vi "art联动采集V4.7(定点后行扫的方案).vi"() -> ()   [LabVIEW 2016]
uses:
  <vilib>/Instr/_visa.llb/VISA Configure Serial Port (Instr).vi
  <vilib>/Utility/file.llb/Write Delimited Spreadsheet (DBL).vi
panel:
  out "x+y 3":dbl=3.0
  in  "分层图查看":bool
  in  "hDevice 2":i32
  in  "逐行扫描":bool
  in  "定位模式":bool
  in  "X终点":dbl
  in  "Y终点":dbl
  in  "高级设置":bool
  in  "Y轴回零速度":dbl=15000.0
  in  "X轴回零速度":dbl=15000.0
  in  "细分设置":dbl=8.0
  in  "等待时间":u32=40
  in  "文件保存":path=path "C:/Users/H301/Desktop/art采集实验数据" caption="保存路径"
  out "行用时（s）":dbl
  out "time（行）":u32
  out "error out":errorcluster caption="错误输出"
  in  "退出扫描(Esc)":bool
  in  "N_Length":i32=16384
  out "M_Length":i32
  out "hDevice":i32=241832032
  out "pulDDR2Length":u32=256
  out "总用时（s）":dbl
  out "毫秒计时值":u32=3586537
  out "数组":dbl[][](array[numeric])=[[58819.77200735986, 88200.32943600747]]
  out "强度图":dbl[][](graph)=[[58819.77200735986, 88200.32943600747]]
  out "judge":dbl
  out "Xloop":dbl
  out "幅频谱":dbl[](graph)
  out "时域谱":dbl[](graph)
  out "错误输出":errorcluster
  in  "启动":bool
  in  "逐点扫描":bool
  in  "X归零":bool
  in  "Y归零":bool
  in  "Y起点":dbl
  in  "Y轴速度":dbl=9000.0
  in  "X轴速度":dbl=9000.0
  out "电机状态":bool
  in  "电机端口":refnum<visa-resource-name>="COM6"
  out "Yloop":dbl=1.0
  out "X扫描范围":dbl=150.0
  out "Y扫描范围":dbl=75.0
  out "Y序":i32
  in  "X起点":dbl
  out "Y(mm)":dbl
  out "x+y 2":dbl=3.0
  in  "Y:":dbl=1.0
  in  "精度":dbl=0.001
  in  "电机急停":bool
  out "X（mm）":dbl
  out "x+y":dbl=1.0
  in  "X:":dbl=1.0
  # "实时坐标"
  # "时域谱"
  # "频域谱"
  # "归零"
  # "扫描区域"
  # "扫描步进(mm)"
  # "X:"
  # "~"
  # "Y:"
  # "~"
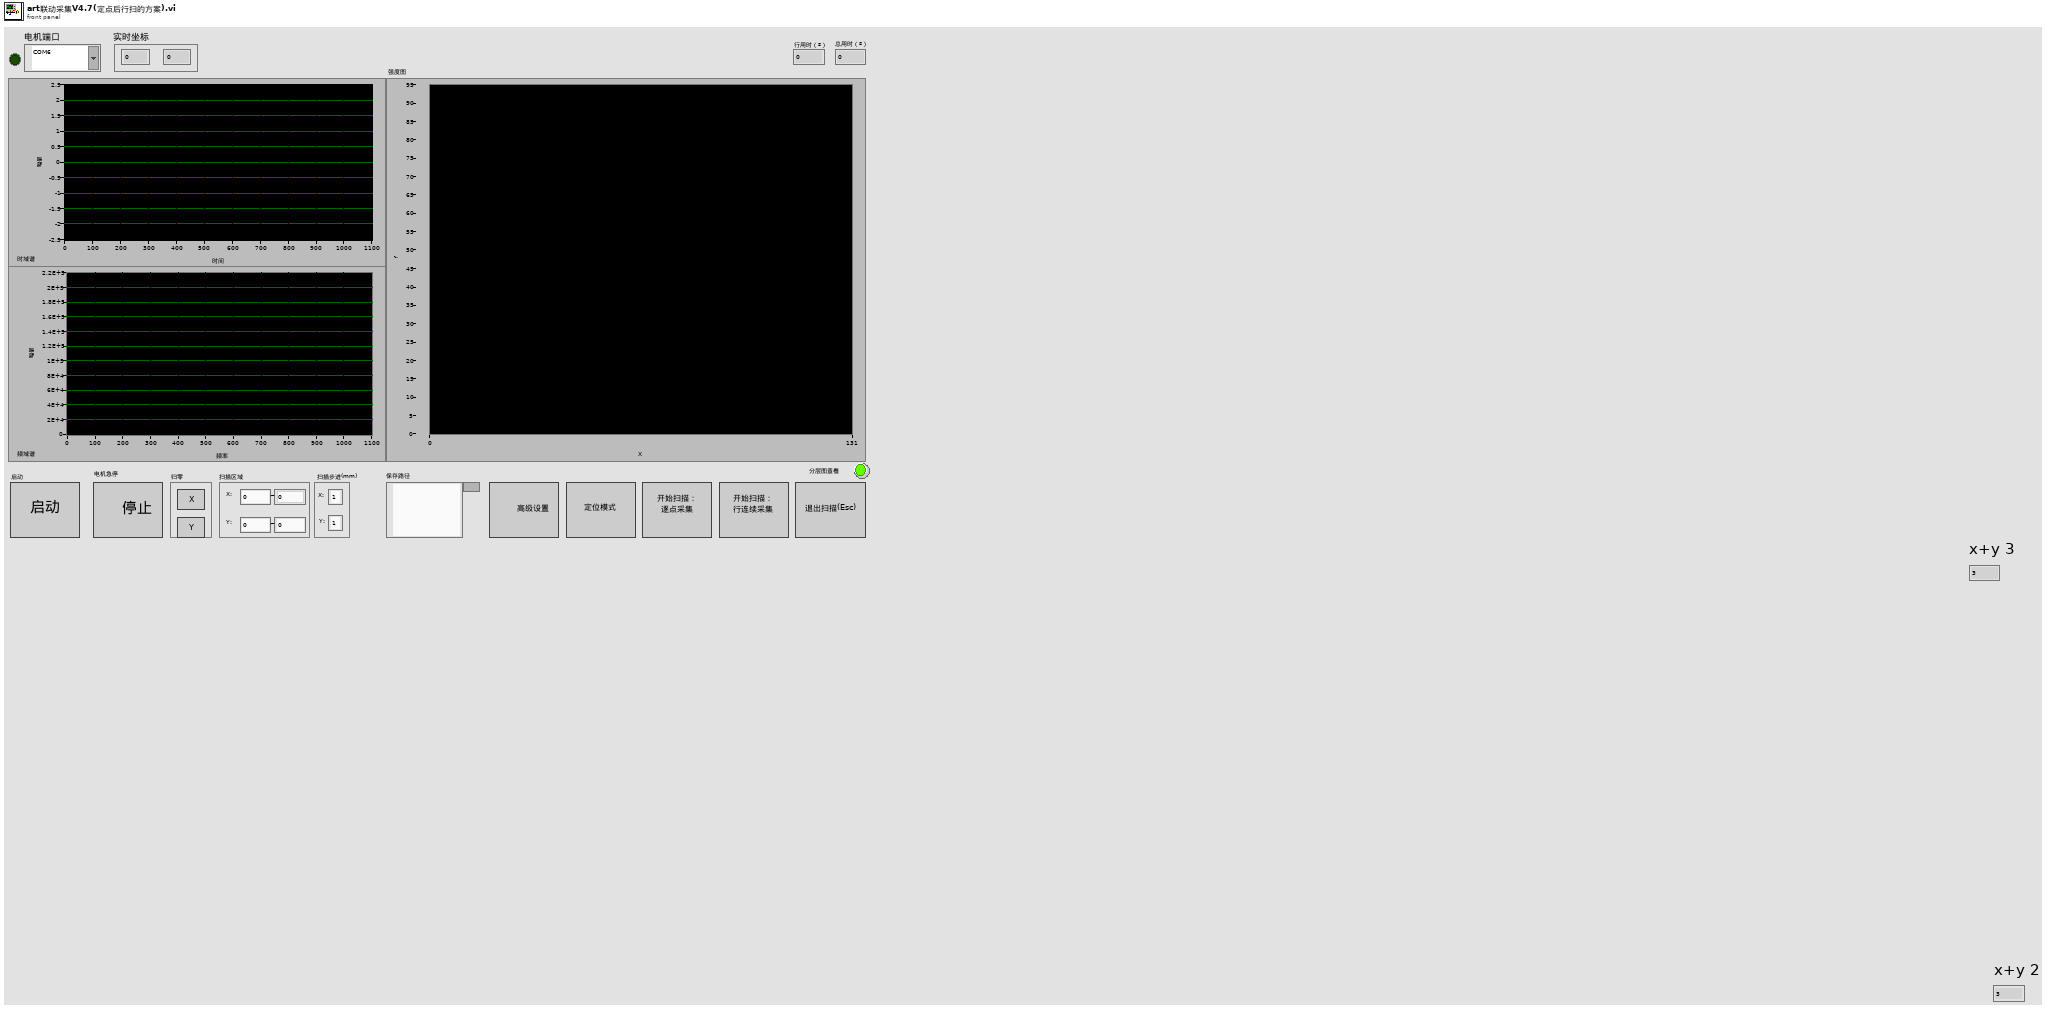
[diagram p1: front panel]
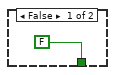
[diagram p2: hidden frame]
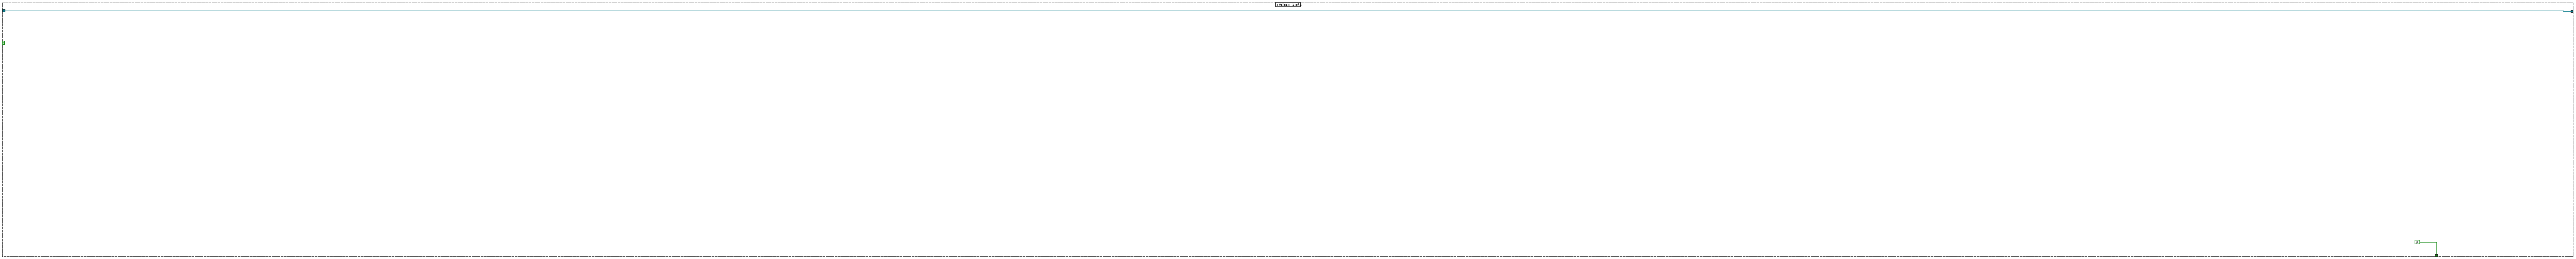
[diagram p3: hidden frame]
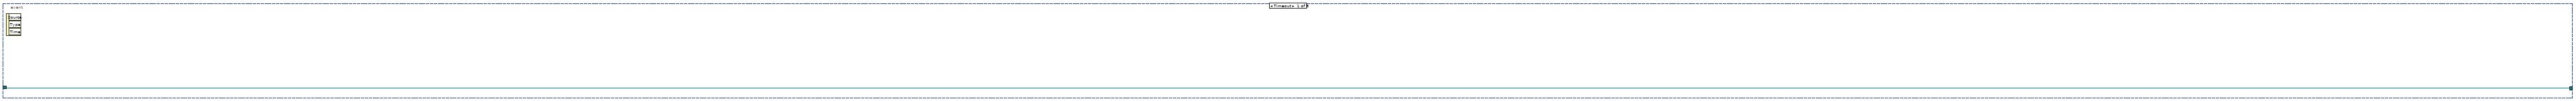
[diagram p4: hidden frame]
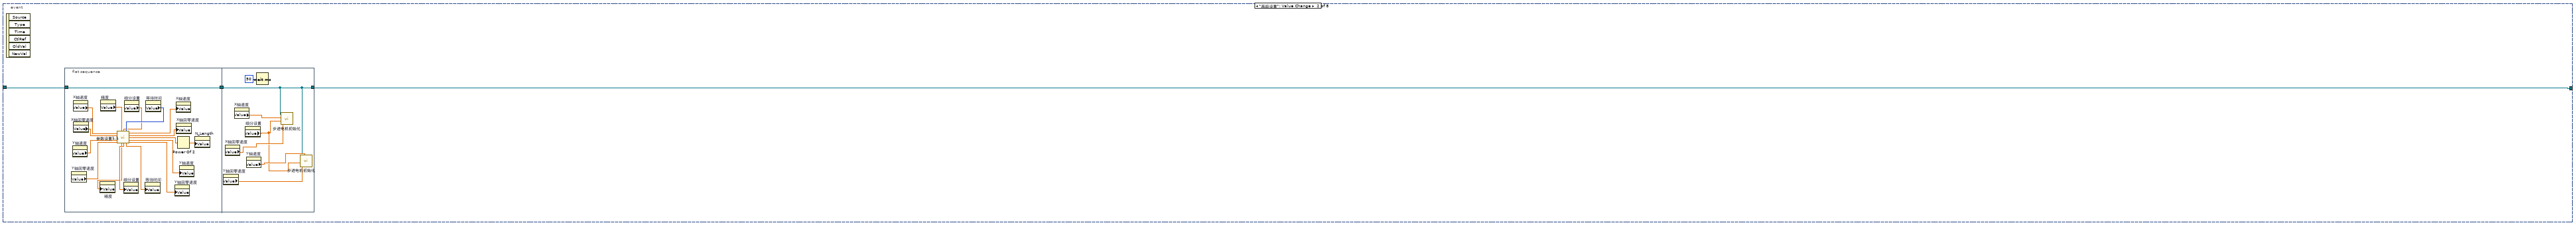
[diagram p5: hidden frame]
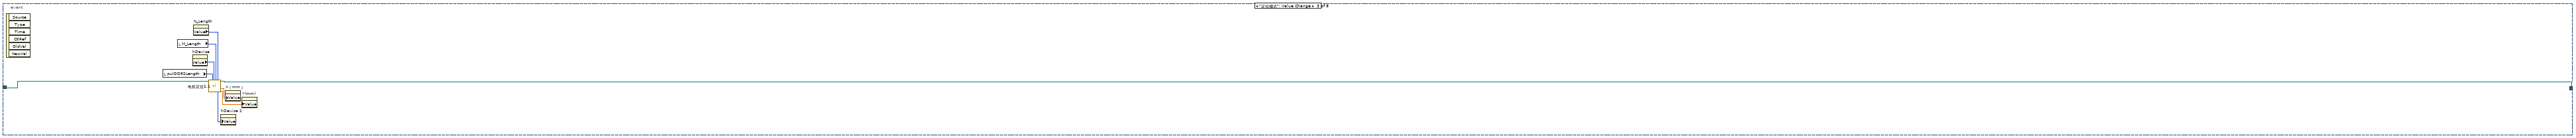
[diagram p6: hidden frame]
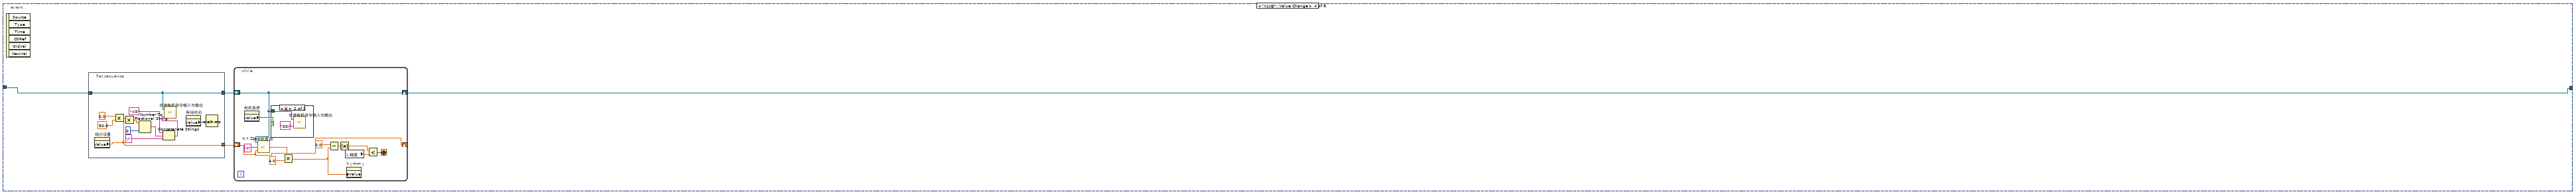
[diagram p7: hidden frame]
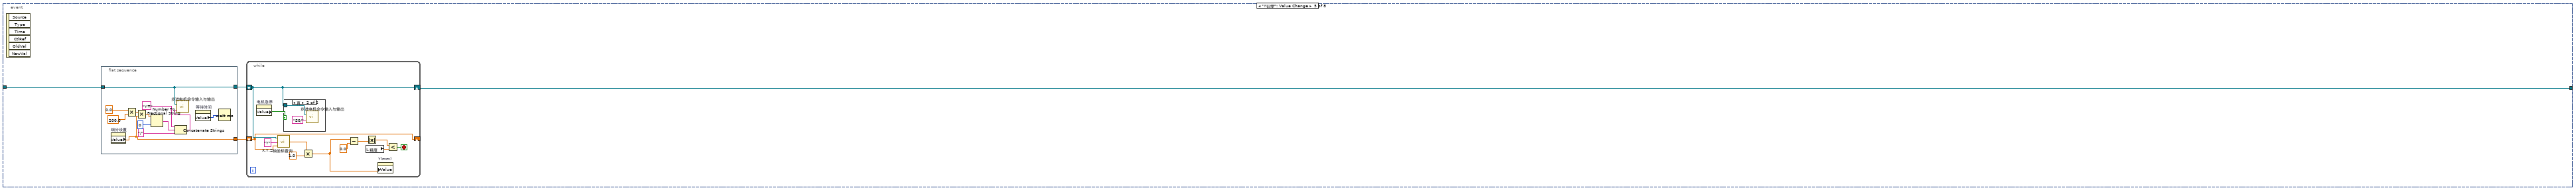
[diagram p9: hidden frame]
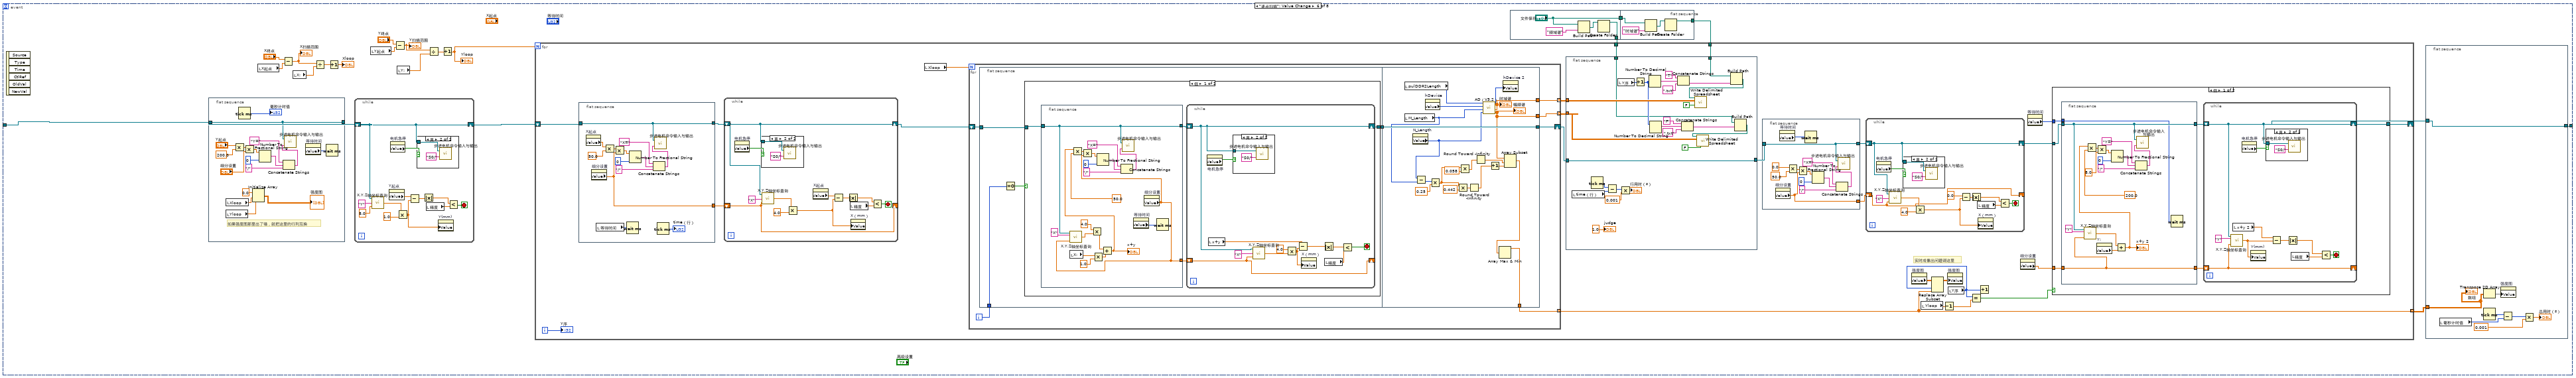
[diagram p11: hidden frame]
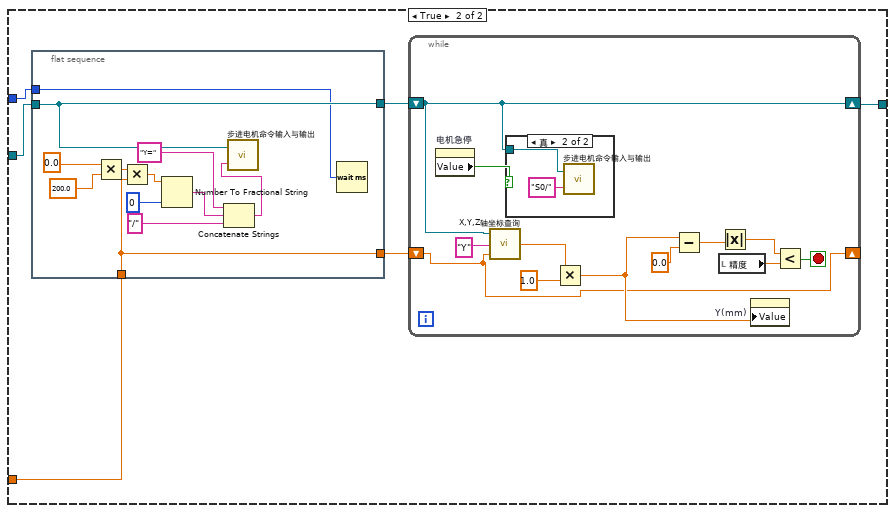
[diagram p16: hidden frame]
diagram:
  n1 = for {
    N: 255 -> [_]
    tunnel: [w10] -> w7 mode=indexing
    i -> [w10]
  }
  n2 = To Unsigned Byte Integer(number=w7) -> (unsigned 8bit integer=w4:u8[])
  n3 = Join Numbers(hi=u16 0, lo=w4) -> ((hi.lo)=w6:u32[])
  n4 = Join Numbers(hi=w4, lo=w4) -> ((hi.lo)=w3:u16[])
  n5 = Join Numbers(hi=w6, lo=w3) -> ((hi.lo)=w2:u64[])
  n6 = property on="强度图" class="IntGraph (严格)"("Color Table"=w2) -> ()  [unwired: 2 in, 2 out]
  n7 = while {
    stop <- w11 stop-if-true
    n8 = case shown="真" "启动" {
      tunnel: [FALSE ("ESC") w20] -> w11
      frame False {
      }
      frame True {
        w33 = 0  # OutClockSource
        w34 = 0  # bClockSourceDir
        w36 = 10000000  # Frequency
        w37 = 0  # ClockSource
        w38 = 0  # TrigLevelVolt
        w26 = 1
        w39 = 0  # TriggerDir
        w40 = 0  # TriggerSource
        w41 = 0  # ATRTriggerChannel
        w42 = 0  # TriggerMode
        w27 = 0  # M_Length
        w43 = 1  # CouplingType
        w44 = 0  # DeviceLgcID
        w54 = u16 0 items=["无", "XON/XOFF", "RTS/CTS", "XON/XOFF & RTS/CTS", "DTR/DSR", "XON/XOFF & DTR/DSR"] ("flow control (0:none)")
        w55 = u16 10 items=["1.0"=10, "1.5"=15, "2.0"=20] ("stop bits (10: 1 bit)")
        # "3"
        # "2"
        # "1"
        n9 = call-poly "VISA Configure Serial Port"("VISA resource name"="电机端口", "baud rate (9600)"=u32 9600, "data bits (8)"=u16 8, "parity (0:none)"=enum16{"None", "Odd", "Even", "Mark", "Space"}."None", "stop bits (10: 1 bit)"=w55, "flow control (0:none)"=w54) -> ("VISA resource name out"=w46:refnum<visa-resource-name>, "error out"=→"error out":errorcluster)  [unwired: 1 in, 7 out]
        n10 = Build Array "InputRange"(w26, w26, w26, w26) -> (w25:i32[])
        n11 = dll-call lib="PTH2aabs CUsersH301Desktopart闭环扫描程序采集卡控制INFamd64PCI8502_32.dll" fn="PCI8502_CreateDevice" label="CreateDevice"("DeviceLgcID"=w44) -> (w31:i32)  [unwired: 4 in, 2 out]
        n12 = property on="细分设置" class="DigNum (严格)"() -> ("Value"=w19:dbl)  [unwired: 2 in, 2 out]
        n13 = Build Array (concatenate) "InitDeviceAD"(w36, w25, w43, w27, "N_Length", w42, w41, w40, w39, w38, w37, w34, w33) -> (w35:i32[])
        n14 = call "步进电机初始化.vi"("回零速度"="X轴回零速度", "细分设置"=w19, "X轴速度"="X轴速度", "串口通信端口"=w46) -> ()  [unwired: 2 in, 1 out]
        n15 = dll-call lib="PTH2aabs CUsersH301Desktopart闭环扫描程序采集卡控制INFamd64PCI8502_32.dll" fn="PCI8502_GetDDR2Length" label="GetDDR2Length"("hDevice"=w31, "pulDDR2Length"=u32 0) -> ("hDevice"=w30:i32, "pulDDR2Length"=→"pulDDR2Length":u32)  [unwired: 4 in, 2 out]
        n16 = call "步进电机初始化.vi"("Y轴速度"="Y轴速度", "回零速度"="Y轴回零速度", "细分设置"=w19, "串口通信端口"=w46) -> ()  [unwired: 2 in, 1 out]
        n17 = call "步进电机命令输入与输出.vi"("输入字符串"="?R/", "串口通信端口"=w46) -> ("返回字符串"=w51:string)
        n18 = dll-call lib="PTH2aabs CUsersH301Desktopart闭环扫描程序采集卡控制INFamd64PCI8502_32.dll" fn="PCI8502_InitDeviceAD" label="InitDeviceAD"("hDevice"=w30, "pADPara"=w35) -> ("hDevice"=→"hDevice":i32)  [unwired: 5 in, 2 out]
        n19 = String Subset(string=w51, offset (0)=0 ("偏移量(0)"), length (rest)=2 ("长度（剩余）")) -> (substring=w48:string)
        n20 = Equal?(x=w48, y="OK") -> (x = y?=w45:bool)
        "电机状态" <- w45
        n21 = case shown="真" w45 {
          tunnel: w46 -> [w61 w64]
          tunnel: [w61 w62] -> w21
          tunnel: [FALSE ("ESC") w63] -> w20
          frame False {
          }
          frame True {
            n22 = while {
              tunnel: ["退出扫描(Esc)"] -> w63
              shift-right: [w65] -> w62
              shift-left: w64 -> [w70]
              stop <- "退出扫描(Esc)" stop-if-true
              n23 = property on="高级设置" class="Bool"("Visible"=TRUE ("可见")) -> ()  [unwired: 2 in, 2 out]
              n24 = property on="定位模式" class="Bool"("Visible"=TRUE ("可见")) -> ()  [unwired: 2 in, 2 out]
              n25 = event shown="[6] \"逐行扫描\": 值改变" {
                selector: _ -> [_ _ _ _ _ _ _ _]
                dyn-events: _ -> [_ _ _ _ _ _ _ _]
                timeout: 1 -> [_ _ _ _ _ _ _ _]
                tunnel: w70 -> [w71 w74 w107 w111 w141 w188 w477 w725]
                tunnel: [w71 w73 w106 w109 w139 w182 w481 w724] -> w65
                event Timeout {
                  n26 = event-data() -> ()  [unwired: 1 in, 3 out]
                }
                event "高级设置": Value Change {
                  n27 = event-data() -> ()  [unwired: 1 in, 6 out]
                  n28 = flat-sequence {
                    tunnel: w74 -> [w77]
                    tunnel: [w77] -> w72
                    tunnel: [w93] -> w73
                    tunnel: w72 -> [w93]
                    frame #0 {
                      n29 = property on="Y轴回零速度" class="DigNum (严格)"() -> ("Value"=w81:dbl)  [unwired: 2 in, 2 out]
                      n30 = property on="Y轴速度" class="DigNum (严格)"() -> ("Value"=w80:dbl)  [unwired: 2 in, 2 out]
                      n31 = property on="X轴速度" class="DigNum (严格)"() -> ("Value"=w78:dbl)  [unwired: 2 in, 2 out]
                      n32 = property on="X轴回零速度" class="DigNum (严格)"() -> ("Value"=w79:dbl)  [unwired: 2 in, 2 out]
                      n33 = property on="精度" class="DigNum (严格)"() -> ("Value"=w85:dbl)  [unwired: 2 in, 2 out]
                      n34 = property on="细分设置" class="DigNum (严格)"() -> ("Value"=w86:dbl)  [unwired: 2 in, 2 out]
                      n35 = property on="等待时间" class="DigNum (严格)"() -> ("Value"=w87:u32)  [unwired: 2 in, 2 out]
                      n36 = call "参数设置1.1.vi"("X轴速度"=w78, "精度"=w85, "细分设置"=w86, "等待时间"=w87, "X轴回零速度"=w79, "Y轴速度"=w80, "Y轴回零速度"=w81) -> ("X轴速度"=w88:dbl, "X轴回零速度"=w89:dbl, "采样阶"=w75:dbl, "Y轴速度"=w90:dbl, "精度"=w82:dbl, "细分设置"=w83:dbl, "等待时间"=w84:dbl, "Y轴回零速度"=w91:dbl)  [unwired: 1 in]
                      n37 = property on="精度" class="DigNum (严格)"("Value"=w82) -> ()  [unwired: 2 in, 2 out]
                      n38 = property on="细分设置" class="DigNum (严格)"("Value"=w83) -> ()  [unwired: 2 in, 2 out]
                      n39 = property on="等待时间" class="DigNum (严格)"("Value"=w84) -> ()  [unwired: 2 in, 2 out]
                      n40 = property on="Y轴回零速度" class="DigNum (严格)"("Value"=w91) -> ()  [unwired: 2 in, 2 out]
                      n41 = property on="X轴速度" class="DigNum (严格)"("Value"=w88) -> ()  [unwired: 2 in, 2 out]
                      n42 = property on="X轴回零速度" class="DigNum (严格)"("Value"=w89) -> ()  [unwired: 2 in, 2 out]
                      n43 = Power Of 2(x=w75) -> (2^x=w76:dbl)
                      n44 = property on="Y轴速度" class="DigNum (严格)"("Value"=w90) -> ()  [unwired: 2 in, 2 out]
                      n45 = property on="N_Length" class="DigNum (严格)"("Value"=w76) -> ()  [unwired: 2 in, 2 out]
                    }
                    frame #1 {
                      n46 = property on="Y轴回零速度" class="DigNum (严格)"() -> ("Value"=w97:dbl)  [unwired: 2 in, 2 out]
                      n47 = property on="X轴回零速度" class="DigNum (严格)"() -> ("Value"=w96:dbl)  [unwired: 2 in, 2 out]
                      n48 = property on="X轴速度" class="DigNum (严格)"() -> ("Value"=w95:dbl)  [unwired: 2 in, 2 out]
                      n49 = property on="细分设置" class="DigNum (严格)"() -> ("Value"=w94:dbl)  [unwired: 2 in, 2 out]
                      n50 = property on="Y轴速度" class="DigNum (严格)"() -> ("Value"=w98:dbl)  [unwired: 2 in, 2 out]
                      n51 = Wait (ms)(milliseconds to wait=u32 50 ("等待时间（毫秒）")) -> ()  [unwired: 1 out]
                      n52 = call "步进电机初始化.vi"("回零速度"=w96, "细分设置"=w94, "X轴速度"=w95, "串口通信端口"=w93) -> ()  [unwired: 2 in, 1 out]
                      n53 = call "步进电机初始化.vi"("Y轴速度"=w98, "回零速度"=w97, "细分设置"=w94, "串口通信端口"=w93) -> ()  [unwired: 2 in, 1 out]
                    }
                  }
                }
                event "定位模式": Value Change {
                  n54 = event-data() -> ()  [unwired: 1 in, 6 out]
                  n55 = local read "pulDDR2Length"() -> (w103:u32)
                  n56 = local read "M_Length"() -> (w101:i32)
                  n57 = property on="hDevice" class="DigNum (严格)"() -> ("Value"=w102:i32)  [unwired: 2 in, 2 out]
                  n58 = property on="N_Length" class="DigNum (严格)"() -> ("Value"=w100:i32)  [unwired: 2 in, 2 out]
                  n59 = call "电机定位1.1.vi"("VISA I"=w107, "pulDDR2Length"=w103, "hDevice"=w102, "M-length"=w101, "N-length"=w100) -> ("hDevice out"=w99:i32, "VISA O"=w106:refnum<visa-resource-name>, "X"=w105:dbl, "Y"=w104:dbl)  [unwired: 11 in]
                  n60 = property on="hDevice 2" class="DigNum (严格)"("Value"=w99) -> ()  [unwired: 2 in, 2 out]
                  n61 = property on="X（mm）" class="DigNum (严格)"("Value"=w105) -> ()  [unwired: 2 in, 2 out]
                  n62 = property on="Y(mm)" class="DigNum (严格)"("Value"=w104) -> ()  [unwired: 2 in, 2 out]
                }
                event "X归零": Value Change {
                  n63 = event-data() -> ()  [unwired: 1 in, 6 out]
                  n64 = flat-sequence {
                    tunnel: w111 -> [w115]
                    tunnel: [w115] -> w110
                    tunnel: [w112] -> w108
                    frame #0 {
                      n65 = property on="细分设置" class="DigNum (严格)"() -> ("Value"=w112:dbl)  [unwired: 2 in, 2 out]
                      n66 = Multiply(x=0.0, y=50.0) -> (x*y=w118:dbl)
                      n67 = Multiply(x=w118, y=w112) -> (x*y=w123:dbl)
                      n68 = Number To Fractional String(number=w123, precision (6)=i16 0 ("精度(6)")) -> (F-format string=w121:string)  [unwired: 2 out]
                      n69 = Concatenate Strings("X=" ("字符串"), w121, "/" ("字符串")) -> (w116:string)
                      n70 = call "步进电机命令输入与输出.vi"("输入字符串"=w116, "串口通信端口"=w115) -> ()  [unwired: 1 out]
                      n71 = property on="等待时间" class="DigNum (严格)"() -> ("Value"=w113:u32)  [unwired: 2 in, 2 out]
                      n72 = Wait (ms)(milliseconds to wait=w113) -> ()  [unwired: 1 out]
                    }
                  }
                  n73 = while {
                    shift-right: [w125] -> w109
                    shift-left: w110 -> [w125]
                    shift-right: [w124] -> _
                    shift-left: w108 -> [w124]
                    stop <- w131 stop-if-true
                    n74 = property on="电机急停" class="Bool (严格)"() -> ("Value"=w132:bool)  [unwired: 2 in, 2 out]
                    n75 = call "X,Y,Z轴坐标查询.vi"("细分设置"=w124, "查询坐标轴"="X", "串口通信端口"=w125) -> ("坐标(mm)"=w133:dbl)
                    n76 = case shown="真" w132 {
                      tunnel: w125 -> [_ w136]
                      frame False {
                      }
                      frame True {
                        n77 = call "步进电机命令输入与输出.vi"("输入字符串"="S0/", "串口通信端口"=w136) -> ()  [unwired: 1 out]
                      }
                    }
                    n78 = Multiply(x=w133, y=4.0 ("x")) -> (x*y=w129:dbl)
                    n79 = Subtract(x=0.0, y=w129) -> (x-y=w128:dbl)
                    n80 = Absolute Value(x=w128) -> (abs(x)=w127:dbl)
                    n81 = local read "精度"() -> (w130:dbl)
                    n82 = property on="X（mm）" class="DigNum (严格)"("Value"=w129) -> ()  [unwired: 2 in, 2 out]
                    n83 = Less?(x=w127, y=w130) -> (x < y?=w131:bool)
                  }
                }
                event "Y归零": Value Change {
                  n84 = event-data() -> ()  [unwired: 1 in, 6 out]
                  n85 = flat-sequence {
                    tunnel: w141 -> [w145]
                    tunnel: [w145] -> w140
                    tunnel: [w142] -> w138
                    frame #0 {
                      n86 = property on="细分设置" class="DigNum (严格)"() -> ("Value"=w142:dbl)  [unwired: 2 in, 2 out]
                      n87 = Multiply(x=0.0, y=200.0) -> (x*y=w148:dbl)
                      n88 = Multiply(x=w148, y=w142) -> (x*y=w153:dbl)
                      n89 = Number To Fractional String(number=w153, precision (6)=i16 0 ("精度(6)")) -> (F-format string=w151:string)  [unwired: 2 out]
                      n90 = Concatenate Strings("Y=" ("字符串"), w151, "/" ("字符串")) -> (w146:string)
                      n91 = call "步进电机命令输入与输出.vi"("输入字符串"=w146, "串口通信端口"=w145) -> ()  [unwired: 1 out]
                      n92 = property on="等待时间" class="DigNum (严格)"() -> ("Value"=w143:u32)  [unwired: 2 in, 2 out]
                      n93 = Wait (ms)(milliseconds to wait=w143) -> ()  [unwired: 1 out]
                    }
                  }
                  n94 = while {
                    shift-right: [w155] -> w139
                    shift-left: w140 -> [w155]
                    shift-right: [w154] -> _
                    shift-left: w138 -> [w154]
                    stop <- w161 stop-if-true
                    n95 = property on="电机急停" class="Bool (严格)"() -> ("Value"=w162:bool)  [unwired: 2 in, 2 out]
                    n96 = call "X,Y,Z轴坐标查询.vi"("细分设置"=w154, "查询坐标轴"="Y", "串口通信端口"=w155) -> ("坐标(mm)"=w163:dbl)
                    n97 = case shown="真" w162 {
                      tunnel: w155 -> [_ w166]
                      frame False {
                      }
                      frame True {
                        n98 = call "步进电机命令输入与输出.vi"("输入字符串"="S0/", "串口通信端口"=w166) -> ()  [unwired: 1 out]
                      }
                    }
                    n99 = Multiply(x=w163, y=1.0 ("x")) -> (x*y=w159:dbl)
                    n100 = Subtract(x=w159, y=0.0 ("x")) -> (x-y=w157:dbl)
                    n101 = local read "精度"() -> (w160:dbl)
                    n102 = Absolute Value(x=w157) -> (abs(x)=w156:dbl)
                    n103 = property on="Y(mm)" class="DigNum (严格)"("Value"=w159) -> ()  [unwired: 2 in, 2 out]
                    n104 = Less?(x=w156, y=w160) -> (x < y?=w161:bool)
                  }
                }
                event "逐点扫描": Value Change {
                  n105 = event-data() -> ()  [unwired: 1 in, 6 out]
                  n106 = flat-sequence {
                    tunnel: w188 -> [w213]
                    tunnel: [w213] -> w178
                    frame #0 {
                      # "如果强度图那里出了错，就把这里的行列互换"
                      n107 = local read "Xloop"() -> (w208:dbl)
                      n108 = local read "Yloop"() -> (w207:dbl)
                      n109 = Multiply(x="Y起点", y=200.0) -> (x*y=w216:dbl)
                      n110 = Tick Count (ms)() -> (millisecond timer value=→"毫秒计时值":u32)
                      n111 = Multiply(x=w216, y="细分设置") -> (x*y=w221:dbl)
                      n112 = Initialize Array(0.0 ("元素"), w208, w207) -> (→"强度图":dbl[][])
                      n113 = Number To Fractional String(number=w221, precision (6)=i16 0 ("精度(6)")) -> (F-format string=w219:string)  [unwired: 2 out]
                      n114 = Concatenate Strings("Y=" ("字符串"), w219, "/" ("字符串")) -> (w214:string)
                      n115 = call "步进电机命令输入与输出.vi"("输入字符串"=w214, "串口通信端口"=w213) -> ()  [unwired: 1 out]
                      n116 = property on="等待时间" class="DigNum (严格)"() -> ("Value"=w205:u32)  [unwired: 2 in, 2 out]
                      n117 = Wait (ms)(milliseconds to wait=w205) -> ()  [unwired: 1 out]
                    }
                  }
                  n118 = local read "X起点"() -> (w174:dbl)
                  n119 = Subtract(x="X终点", y=w174) -> (x-y=w173:dbl)
                  "X扫描范围" <- w173
                  n120 = local read "X:"() -> (w181:dbl)
                  n121 = Divide(x=w173, y=w181) -> (x/y=w179:dbl)
                  n122 = Increment(x=w179) -> (x+1=→"Xloop":dbl)
                  n123 = while {
                    shift-right: [w222] -> w170
                    shift-left: w178 -> [w222]
                    stop <- w227 stop-if-true
                    n124 = call "X,Y,Z轴坐标查询.vi"("细分设置"=8.0, "查询坐标轴"="Y", "串口通信端口"=w222) -> ("坐标(mm)"=w229:dbl)
                    n125 = property on="Y起点" class="DigNum (严格)"() -> ("Value"=w231:dbl)  [unwired: 2 in, 2 out]
                    n126 = property on="电机急停" class="Bool (严格)"() -> ("Value"=w228:bool)  [unwired: 2 in, 2 out]
                    n127 = Multiply(x=w229, y=1.0 ("x")) -> (x*y=w225:dbl)
                    n128 = Subtract(x=w231, y=w225) -> (x-y=w224:dbl)
                    n129 = case shown="真" w228 {
                      tunnel: w222 -> [_ w234]
                      frame False {
                      }
                      frame True {
                        n130 = call "步进电机命令输入与输出.vi"("输入字符串"="S0/", "串口通信端口"=w234) -> ()  [unwired: 1 out]
                      }
                    }
                    n131 = Absolute Value(x=w224) -> (abs(x)=w223:dbl)
                    n132 = local read "精度"() -> (w226:dbl)
                    n133 = property on="Y(mm)" class="DigNum (严格)"("Value"=w225) -> ()  [unwired: 2 in, 2 out]
                    n134 = Less?(x=w223, y=w226) -> (x < y?=w227:bool)
                  }
                  n135 = local read "Y起点"() -> (w176:dbl)
                  n136 = Subtract(x="Y终点", y=w176) -> (x-y=w172:dbl)
                  "Y扫描范围" <- w172
                  n137 = local read "Y:"() -> (w187:dbl)
                  n138 = Divide(x=w172, y=w187) -> (x/y=w186:dbl)
                  n139 = Increment(x=w186) -> (x+1=w185:dbl)
                  "Yloop" <- w185
                  n140 = for {
                    N: w185 -> [_]
                    shift-right: [w258] -> w184
                    shift-left: w170 -> [w238]
                    tunnel: [w240] -> w183 mode=indexing
                    tunnel: w168 -> [w244]
                    tunnel: w171 -> [w243]
                    i -> [w259]
                    # "实时成像出问题调这里"
                    n141 = flat-sequence {
                      tunnel: w238 -> [w316]
                      tunnel: [w316] -> w257
                      tunnel: [w314] -> w248
                      frame #0 {
                        n142 = property on="X起点" class="DigNum (严格)"() -> ("Value"=w312:dbl)  [unwired: 2 in, 2 out]
                        n143 = property on="细分设置" class="DigNum (严格)"() -> ("Value"=w314:dbl)  [unwired: 2 in, 2 out]
                        n144 = local read "等待时间"() -> (w313:u32)
                        n145 = Multiply(x=w312, y=50.0) -> (x*y=w319:dbl)
                        n146 = Multiply(x=w319, y=w314) -> (x*y=w324:dbl)
                        n147 = Wait (ms)(milliseconds to wait=w313) -> ()  [unwired: 1 out]
                        n148 = Number To Fractional String(number=w324, precision (6)=i16 0 ("精度(6)")) -> (F-format string=w322:string)  [unwired: 2 out]
                        n149 = Concatenate Strings("X=" ("字符串"), w322, "/" ("字符串")) -> (w317:string)
                        n150 = call "步进电机命令输入与输出.vi"("输入字符串"=w317, "串口通信端口"=w316) -> ()  [unwired: 1 out]
                        n151 = Tick Count (ms)() -> (millisecond timer value=→"time（行）":u32)
                      }
                    }
                    n152 = while {
                      shift-right: [w326] -> w236
                      shift-left: w257 -> [w326]
                      shift-right: [w325] -> _
                      shift-left: w248 -> [w325]
                      stop <- w331 stop-if-true
                      n153 = property on="电机急停" class="Bool (严格)"() -> ("Value"=w332:bool)  [unwired: 2 in, 2 out]
                      n154 = case shown="真" w332 {
                        tunnel: w326 -> [_ w337]
                        frame False {
                        }
                        frame True {
                          n155 = call "步进电机命令输入与输出.vi"("输入字符串"="S0/", "串口通信端口"=w337) -> ()  [unwired: 1 out]
                        }
                      }
                      n156 = call "X,Y,Z轴坐标查询.vi"("细分设置"=w325, "查询坐标轴"="X", "串口通信端口"=w326) -> ("坐标(mm)"=w333:dbl)
                      n157 = Multiply(x=w333, y=4.0 ("x")) -> (x*y=w329:dbl)
                      n158 = property on="X起点" class="DigNum (严格)"() -> ("Value"=w335:dbl)  [unwired: 2 in, 2 out]
                      n159 = Subtract(x=w335, y=w329) -> (x-y=w328:dbl)
                      n160 = Absolute Value(x=w328) -> (abs(x)=w327:dbl)
                      n161 = local read "精度"() -> (w330:dbl)
                      n162 = property on="X（mm）" class="DigNum (严格)"("Value"=w329) -> ()  [unwired: 2 in, 2 out]
                      n163 = Less?(x=w327, y=w330) -> (x < y?=w331:bool)
                    }
                    n164 = local read "Xloop"() -> (w249:dbl)
                    n165 = for {
                      N: w249 -> [_]
                      shift-right: [w410] -> w237
                      shift-left: w236 -> [w405]
                      tunnel: [w409] -> w256 mode=indexing
                      tunnel: [w408] -> w255 mode=indexing
                      tunnel: [w407] -> w240 mode=indexing
                      i -> [w406]
                      n166 = flat-sequence {
                        tunnel: w405 -> [w415]
                        tunnel: [w414] -> w411
                        tunnel: w406 -> [w412]
                        tunnel: [w473] -> w410
                        tunnel: w411 -> [w473]
                        tunnel: [w472] -> w409
                        tunnel: [w471] -> w408
                        tunnel: [w469] -> w407
                        frame #0 {
                          n167 = Equal To 0?(x=w412) -> (x = 0?=w413:bool)
                          n168 = case shown="假" w413 {
                            tunnel: w415 -> [w418 w453]
                            tunnel: [w417 w453] -> w414
                            frame False {
                              n169 = flat-sequence {
                                tunnel: w418 -> [w428]
                                tunnel: [w428] -> w419
                                tunnel: [w420] -> w416
                                frame #0 {
                                n170 = local read "X:"() -> (w422:dbl)
                                n171 = Multiply(x=w422, y=1.0 ("x")) -> (x*y=w427:dbl)
                                n172 = property on="等待时间" class="DigNum (严格)"() -> ("Value"=w421:u32)  [unwired: 2 in, 2 out]
                                n173 = property on="细分设置" class="DigNum (严格)"() -> ("Value"=w420:dbl)  [unwired: 2 in, 2 out]
                                n174 = call "X,Y,Z轴坐标查询.vi"("细分设置"=w420, "查询坐标轴"="X", "串口通信端口"=w428) -> ("坐标(mm)"=w424:dbl)
                                n175 = Multiply(x=4.0, y=w424) -> (x*y=w423:dbl)
                                n176 = Add(x=w423, y=w427) -> (x+y=w430:dbl)
                                "x+y" <- w430
                                n177 = Multiply(x=w430, y=50.0) -> (x*y=w433:dbl)
                                n178 = Multiply(x=w433, y=w420) -> (x*y=w438:dbl)
                                n179 = Number To Fractional String(number=w438, precision (6)=i16 0 ("精度(6)")) -> (F-format string=w436:string)  [unwired: 2 out]
                                n180 = Concatenate Strings("X=" ("字符串"), w436, "/" ("字符串")) -> (w431:string)
                                n181 = call "步进电机命令输入与输出.vi"("输入字符串"=w431, "串口通信端口"=w428) -> ()  [unwired: 1 out]
                                n182 = Wait (ms)(milliseconds to wait=w421) -> ()  [unwired: 1 out]
                                }
                              }
                              n183 = while {
                                shift-right: [w448] -> w417
                                shift-left: w419 -> [w448]
                                shift-right: [w439] -> _
                                shift-left: w416 -> [w439]
                                stop <- w447 stop-if-true
                                n184 = property on="电机急停" class="Bool (严格)"() -> ("Value"=w445:bool)  [unwired: 2 in, 2 out]
                                n185 = local read "x+y"() -> (w449:dbl)
                                n186 = case shown="真" w445 {
                                tunnel: w448 -> [_ w451]
                                frame False {
                                }
                                frame True {
                                n187 = call "步进电机命令输入与输出.vi"("输入字符串"="S0/", "串口通信端口"=w451) -> ()  [unwired: 1 out]
                                }
                                }
                                n188 = call "X,Y,Z轴坐标查询.vi"("细分设置"=w439, "查询坐标轴"="X", "串口通信端口"=w448) -> ("坐标(mm)"=w443:dbl)
                                n189 = Multiply(x=4.0, y=w443) -> (x*y=w442:dbl)
                                n190 = Subtract(x=w449, y=w442) -> (x-y=w441:dbl)
                                n191 = property on="X（mm）" class="DigNum (严格)"("Value"=w442) -> ()  [unwired: 2 in, 2 out]
                                n192 = Absolute Value(x=w441) -> (abs(x)=w440:dbl)
                                n193 = local read "精度"() -> (w444:dbl)
                                n194 = Less?(x=w440, y=w444) -> (x < y?=w447:bool)
                              }
                            }
                            frame True {
                            }
                          }
                        }
                        frame #1 {
                          n195 = local read "pulDDR2Length"() -> (w468:u32)
                          n196 = local read "M_Length"() -> (w467:i32)
                          n197 = property on="N_Length" class="DigNum (严格)"() -> ("Value"=w456:i32)  [unwired: 2 in, 2 out]
                          n198 = Subtract(x=w456, y=w467) -> (x-y=w465:i32)
                          n199 = property on="hDevice" class="DigNum (严格)"() -> ("Value"=w454:i32)  [unwired: 2 in, 2 out]
                          n200 = Multiply(x=w465, y=0.25) -> (x*y=w458:dbl)
                          n201 = Multiply(x=w458, y=0.442) -> (x*y=w460:dbl)
                          n202 = Multiply(x=w458, y=0.058) -> (x*y=w462:dbl)
                          n203 = Round Toward -Infinity(1:w460) -> (0:w457:dbl)
                          n204 = Round Toward -Infinity(1:w462) -> (0:w461:dbl)
                          n205 = call "AD（V3.2）.vi"("N-length"=w456, "M-length"=w467, "hDevice"=w454, "pulDDR2Length"=w468) -> ("幅频谱"=w471:dbl[], "时域谱"=w472:dbl[], "hDevice out"=w455:i32)  [unwired: 5 in]
                          "时域谱" <- w472
                          "幅频谱" <- w471
                          n206 = Increment(x=w457) -> (x+1=w464:dbl)
                          n207 = property on="hDevice 2" class="DigNum (严格)"("Value"=w455) -> ()  [unwired: 2 in, 2 out]
                          n208 = Array Subset(array=w471, index=w461, length=w464) -> (w470:dbl[])
                          n209 = Array Max & Min(array=w470) -> (max value=w469:dbl)  [unwired: 3 out]
                        }
                      }
                    }
                    n210 = flat-sequence {
                      tunnel: w255 -> [w293]
                      tunnel: w256 -> [w301]
                      tunnel: w237 -> [w310]
                      tunnel: [w310] -> w251
                      tunnel: w244 -> [w288]
                      tunnel: w243 -> [w287]
                      frame #0 {
                        n211 = local read "time（行）"() -> (w309:u32)
                        n212 = Tick Count (ms)() -> (millisecond timer value=w305:u32)
                        n213 = Subtract(x=w305, y=w309) -> (x-y=w308:u32)
                        n214 = local read "Y序"() -> (w289:i32)
                        n215 = Multiply(x=w308, y=0.001) -> (x*y=→"行用时（s）":dbl)
                        n216 = Increment(x=w289) -> (x+1=w290:i32)
                        n217 = Number To Decimal String(number=w290) -> (decimal integer string=w299:string)  [unwired: 1 in]
                        n218 = Number To Decimal String(number=w290) -> (decimal integer string=w298:string)  [unwired: 1 in]
                        n219 = Concatenate Strings("T" ("字符串"), w299, ".txt" ("字符串")) -> (w302:string)
                        n220 = Concatenate Strings("F" ("字符串"), w298, ".txt" ("字符串")) -> (w296:string)
                        n221 = Build Path(base path=w288, name or relative path=w302) -> (appended path=w304:path)
                        n222 = call-poly <vilib>:"Write Delimited Spreadsheet.vi"("file path (dialog if empty)"=w304, "2D data"=w301, "transpose? (no:F)"=FALSE) -> ()  [unwired: 11 in, 2 out]
                        n223 = Build Path(base path=w287, name or relative path=w296) -> (appended path=w294:path)
                        n224 = call-poly <vilib>:"Write Delimited Spreadsheet.vi"("file path (dialog if empty)"=w294, "2D data"=w293, "transpose? (no:F)"=FALSE) -> ()  [unwired: 11 in, 2 out]
                        "judge" <- 1.0
                      }
                    }
                    n225 = flat-sequence {
                      tunnel: w251 -> [w264]
                      tunnel: [w264] -> w252
                      tunnel: [w262] -> w247
                      frame #0 {
                        n226 = property on="细分设置" class="DigNum (严格)"() -> ("Value"=w262:dbl)  [unwired: 2 in, 2 out]
                        n227 = property on="等待时间" class="DigNum (严格)"() -> ("Value"=w261:u32)  [unwired: 2 in, 2 out]
                        n228 = Multiply(x=0.0, y=50.0) -> (x*y=w267:dbl)
                        n229 = Multiply(x=w267, y=w262) -> (x*y=w272:dbl)
                        n230 = Wait (ms)(milliseconds to wait=w261) -> ()  [unwired: 1 out]
                        n231 = Number To Fractional String(number=w272, precision (6)=i16 0 ("精度(6)")) -> (F-format string=w270:string)  [unwired: 2 out]
                        n232 = Concatenate Strings("X=" ("字符串"), w270, "/" ("字符串")) -> (w265:string)
                        n233 = call "步进电机命令输入与输出.vi"("输入字符串"=w265, "串口通信端口"=w264) -> ()  [unwired: 1 out]
                      }
                    }
                    n234 = while {
                      shift-right: [w274] -> w250
                      shift-left: w252 -> [w274]
                      shift-right: [w273] -> _
                      shift-left: w247 -> [w273]
                      stop <- w280 stop-if-true
                      n235 = property on="电机急停" class="Bool (严格)"() -> ("Value"=w281:bool)  [unwired: 2 in, 2 out]
                      n236 = call "X,Y,Z轴坐标查询.vi"("细分设置"=w273, "查询坐标轴"="X", "串口通信端口"=w274) -> ("坐标(mm)"=w282:dbl)
                      n237 = case shown="真" w281 {
                        tunnel: w274 -> [_ w285]
                        frame False {
                        }
                        frame True {
                          n238 = call "步进电机命令输入与输出.vi"("输入字符串"="S0/", "串口通信端口"=w285) -> ()  [unwired: 1 out]
                        }
                      }
                      n239 = Multiply(x=w282, y=4.0 ("x")) -> (x*y=w278:dbl)
                      n240 = Subtract(x=0.0, y=w278) -> (x-y=w277:dbl)
                      n241 = Absolute Value(x=w277) -> (abs(x)=w276:dbl)
                      n242 = local read "精度"() -> (w279:dbl)
                      n243 = property on="X（mm）" class="DigNum (严格)"("Value"=w278) -> ()  [unwired: 2 in, 2 out]
                      n244 = Less?(x=w276, y=w279) -> (x < y?=w280:bool)
                    }
                    n245 = property on="强度图" class="IntGraph (严格)"() -> ("Value"=w241:dbl[][])  [unwired: 2 in, 2 out]
                    n246 = local read "Yloop"() -> (w253:dbl)
                    n247 = Decrement(x=w253) -> (x-1=w254:dbl)
                    n248 = local read "Y序"() -> (w239:i32)
                    n249 = Replace Array Subset(array=w241, new element=w240, index (col)=w239) -> (w242:dbl[][])  [unwired: 1 in]
                    n250 = property on="强度图" class="IntGraph (严格)"("Value"=w242) -> ()  [unwired: 2 in, 2 out]
                    n251 = Equal?(x=w239, y=w254) -> (x = y?=w260:bool)
                    n252 = Increment(x=w239) -> ()  [unwired: 1 out]
                    n253 = property on="细分设置" class="DigNum (严格)"() -> ("Value"=w245:dbl)  [unwired: 2 in, 2 out]
                    n254 = property on="等待时间" class="DigNum (严格)"() -> ("Value"=w246:u32)  [unwired: 2 in, 2 out]
                    n255 = case shown="假" w260 {
                      tunnel: w250 -> [w344 w376]
                      tunnel: [w342 w377] -> w258
                      tunnel: w246 -> [w340 w374]
                      tunnel: w245 -> [w339 w373]
                      frame False {
                        n256 = flat-sequence {
                          tunnel: w344 -> [w348]
                          tunnel: [w348] -> w343
                          tunnel: [w346] -> w341
                          tunnel: w340 -> [w347]
                          tunnel: w339 -> [w346]
                          frame #0 {
                            n257 = call "X,Y,Z轴坐标查询.vi"("细分设置"=w346, "查询坐标轴"="Y", "串口通信端口"=w348) -> ("坐标(mm)"=w349:dbl)
                            n258 = property on="Y:" class="DigNum (严格)"() -> ("Value"=w345:dbl)  [unwired: 2 in, 2 out]
                            n259 = Add(x=w349, y=w345) -> (x+y=w351:dbl)
                            "x+y 2" <- w351
                            n260 = Multiply(x=w351, y=200.0) -> (x*y=w355:dbl)
                            n261 = Multiply(x=w355, y=8.0 ("细分设置")) -> (x*y=w360:dbl)
                            n262 = Number To Fractional String(number=w360, precision (6)=i16 0 ("精度(6)")) -> (F-format string=w358:string)  [unwired: 2 out]
                            n263 = Concatenate Strings("Y=" ("字符串"), w358, "/" ("字符串")) -> (w353:string)
                            n264 = call "步进电机命令输入与输出.vi"("输入字符串"=w353, "串口通信端口"=w348) -> ()  [unwired: 1 out]
                            n265 = Wait (ms)(milliseconds to wait=w347) -> ()  [unwired: 1 out]
                          }
                        }
                        n266 = while {
                          shift-right: [w362] -> w342
                          shift-left: w343 -> [w362]
                          shift-right: [w361] -> _
                          shift-left: w341 -> [w361]
                          stop <- w368 stop-if-true
                          n267 = call "X,Y,Z轴坐标查询.vi"("细分设置"=w361, "查询坐标轴"="Y", "串口通信端口"=w362) -> ("坐标(mm)"=w366:dbl)
                          n268 = local read "x+y 2"() -> (w369:dbl)
                          n269 = property on="电机急停" class="Bool (严格)"() -> ("Value"=w365:bool)  [unwired: 2 in, 2 out]
                          n270 = property on="Y(mm)" class="DigNum (严格)"("Value"=w366) -> ()  [unwired: 2 in, 2 out]
                          n271 = case shown="真" w365 {
                            tunnel: w362 -> [_ w371]
                            frame False {
                            }
                            frame True {
                              n272 = call "步进电机命令输入与输出.vi"("输入字符串"="S0/", "串口通信端口"=w371) -> ()  [unwired: 1 out]
                            }
                          }
                          n273 = Subtract(x=w369, y=w366) -> (x-y=w364:dbl)
                          n274 = Absolute Value(x=w364) -> (abs(x)=w363:dbl)
                          n275 = local read "精度"() -> (w367:dbl)
                          n276 = Less?(x=w363, y=w367) -> (x < y?=w368:bool)
                        }
                      }
                      frame True {
                        n277 = flat-sequence {
                          tunnel: [w381] -> _
                          tunnel: [w381] -> w378
                          tunnel: w376 -> [w381]
                          tunnel: [w379] -> w375
                          tunnel: w374 -> [w380]
                          tunnel: w373 -> [w379]
                          frame #0 {
                            n278 = Multiply(x=0.0, y=200.0) -> (x*y=w385:dbl)
                            n279 = Multiply(x=w385, y=w379) -> (x*y=w390:dbl)
                            n280 = Number To Fractional String(number=w390, precision (6)=i16 0 ("精度(6)")) -> (F-format string=w388:string)  [unwired: 2 out]
                            n281 = Concatenate Strings("Y=" ("字符串"), w388, "/" ("字符串")) -> (w383:string)
                            n282 = call "步进电机命令输入与输出.vi"("输入字符串"=w383, "串口通信端口"=w381) -> ()  [unwired: 1 out]
                            n283 = Wait (ms)(milliseconds to wait=w380) -> ()  [unwired: 1 out]
                          }
                        }
                        n284 = while {
                          shift-right: [w392] -> w377
                          shift-left: w378 -> [w392]
                          shift-right: [w391] -> _
                          shift-left: w375 -> [w391]
                          stop <- w398 stop-if-true
                          n285 = property on="电机急停" class="Bool (严格)"() -> ("Value"=w399:bool)  [unwired: 2 in, 2 out]
                          n286 = call "X,Y,Z轴坐标查询.vi"("细分设置"=w391, "查询坐标轴"="Y", "串口通信端口"=w392) -> ("坐标(mm)"=w400:dbl)
                          n287 = case shown="真" w399 {
                            tunnel: w392 -> [_ w403]
                            frame False {
                            }
                            frame True {
                              n288 = call "步进电机命令输入与输出.vi"("输入字符串"="S0/", "串口通信端口"=w403) -> ()  [unwired: 1 out]
                            }
                          }
                          n289 = Multiply(x=w400, y=1.0 ("x")) -> (x*y=w396:dbl)
                          n290 = Subtract(x=w396, y=0.0 ("x")) -> (x-y=w394:dbl)
                          n291 = local read "精度"() -> (w397:dbl)
                          n292 = Absolute Value(x=w394) -> (abs(x)=w393:dbl)
                          n293 = property on="Y(mm)" class="DigNum (严格)"("Value"=w396) -> ()  [unwired: 2 in, 2 out]
                          n294 = Less?(x=w393, y=w397) -> (x < y?=w398:bool)
                        }
                      }
                    }
                    "Y序" <- w259
                  }
                  n295 = flat-sequence {
                    tunnel: [w189] -> w171
                    tunnel: ["文件保存"] -> w169
                    tunnel: w169 -> [w194]
                    tunnel: [w193] -> w168
                    frame #0 {
                      n296 = Build Path(base path="文件保存", name or relative path="频域谱" ("名称或相对路径")) -> (appended path=w192:path)
                      n297 = Create Folder(path (use dialog)=w192) -> (created path=w189:path)  [unwired: 2 in, 2 out]
                    }
                    frame #1 {
                      n298 = Build Path(base path=w194, name or relative path="时域谱" ("名称或相对路径")) -> (appended path=w195:path)
                      n299 = Create Folder(path (use dialog)=w195) -> (created path=w193:path)  [unwired: 2 in, 2 out]
                    }
                  }
                  n300 = flat-sequence {
                    tunnel: w184 -> [w199]
                    tunnel: w183 -> [w198]
                    tunnel: [w199] -> w182
                    frame #0 {
                      n301 = local read "毫秒计时值"() -> (w203:u32)
                      n302 = Transpose 2D Array(2D array=w198) -> (transposed array=w197:dbl[][])
                      n303 = Tick Count (ms)() -> (millisecond timer value=w204:u32)
                      n304 = property on="强度图" class="IntGraph (严格)"("Value"=w197) -> ()  [unwired: 2 in, 2 out]
                      n305 = Subtract(x=w204, y=w203) -> (x-y=w200:u32)
                      n306 = Multiply(x=w200, y=0.001) -> (x*y=→"总用时（s）":dbl)
                      "数组" <- w198
                    }
                  }
                }
                event "逐行扫描": Value Change {
                  n307 = event-data() -> ()  [unwired: 1 in, 6 out]
                  n308 = flat-sequence {
                    tunnel: [w540] -> w483
                    tunnel: [w539] -> w479
                    tunnel: w483 -> [w544]
                    tunnel: [w543] -> w482
                    frame #0 {
                      n309 = local read "文件保存"() -> (w540:path)
                      n310 = Build Path(base path=w540, name or relative path="频域谱" ("名称或相对路径")) -> (appended path=w542:path)
                      n311 = Create Folder(path (use dialog)=w542) -> (created path=w539:path)  [unwired: 2 in, 2 out]
                    }
                    frame #1 {
                      n312 = Build Path(base path=w544, name or relative path="时域谱" ("名称或相对路径")) -> (appended path=w545:path)
                      n313 = Create Folder(path (use dialog)=w545) -> (created path=w543:path)  [unwired: 2 in, 2 out]
                    }
                  }
                  n314 = flat-sequence {
                    tunnel: w477 -> [w500]
                    tunnel: [w500] -> w476
                    frame #0 {
                      # "如果强度图那里出了错，就把这里的行列互换"
                      n315 = property on="Y起点" class="DigNum (严格)"() -> ("Value"=w503:dbl)  [unwired: 2 in, 2 out]
                      n316 = property on="细分设置" class="DigNum (严格)"() -> ("Value"=w501:dbl)  [unwired: 2 in, 2 out]
                      n317 = local read "Xloop"() -> (w507:dbl)
                      n318 = local read "Yloop"() -> (w506:dbl)
                      n319 = Multiply(x=w503, y=200.0) -> (x*y=w511:dbl)
                      n320 = Tick Count (ms)() -> (millisecond timer value=w504:u32)
                      n321 = Multiply(x=w511, y=w501) -> (x*y=w516:dbl)
                      n322 = Initialize Array(0.0 ("元素"), w507, w506) -> (w502:dbl[][])
                      n323 = Number To Fractional String(number=w516, precision (6)=i16 0 ("精度(6)")) -> (F-format string=w514:string)  [unwired: 2 out]
                      n324 = property on="毫秒计时值" class="DigNum (严格)"("Value"=w504) -> ()  [unwired: 2 in, 2 out]
                      n325 = property on="强度图" class="IntGraph (严格)"("Value"=w502) -> ()  [unwired: 2 in, 2 out]
                      n326 = Concatenate Strings("Y=" ("字符串"), w514, "/" ("字符串")) -> (w509:string)
                      n327 = call "步进电机命令输入与输出.vi"("输入字符串"=w509, "串口通信端口"=w500) -> ()  [unwired: 1 out]
                      n328 = property on="等待时间" class="DigNum (严格)"() -> ("Value"=w505:u32)  [unwired: 2 in, 2 out]
                      n329 = Wait (ms)(milliseconds to wait=w505) -> ()  [unwired: 1 out]
                    }
                  }
                  n330 = flat-sequence {
                    tunnel: [w496] -> w475
                    frame #0 {
                      n331 = property on="X终点" class="DigNum (严格)"() -> ("Value"=w485:dbl)  [unwired: 2 in, 2 out]
                      n332 = property on="X起点" class="DigNum (严格)"() -> ("Value"=w484:dbl)  [unwired: 2 in, 2 out]
                      n333 = Subtract(x=w485, y=w484) -> (x-y=w489:dbl)
                      n334 = local read "X:"() -> (w488:dbl)
                      n335 = property on="X扫描范围" class="DigNum (严格)"("Value"=w489) -> ()  [unwired: 2 in, 2 out]
                      n336 = Divide(x=w489, y=w488) -> (x/y=w487:dbl)
                      n337 = Increment(x=w487) -> (x+1=w486:dbl)
                      n338 = property on="Xloop" class="DigNum (严格)"("Value"=w486) -> ()  [unwired: 2 in, 2 out]
                    }
                    frame #1 {
                      n339 = property on="Y终点" class="DigNum (严格)"() -> ("Value"=w491:dbl)  [unwired: 2 in, 2 out]
                      n340 = property on="Y起点" class="DigNum (严格)"() -> ("Value"=w490:dbl)  [unwired: 2 in, 2 out]
                      n341 = Subtract(x=w491, y=w490) -> (x-y=w494:dbl)
                      n342 = local read "Y:"() -> (w493:dbl)
                      n343 = property on="Y扫描范围" class="DigNum (严格)"("Value"=w494) -> ()  [unwired: 2 in, 2 out]
                      n344 = Divide(x=w494, y=w493) -> (x/y=w495:dbl)
                      n345 = Increment(x=w495) -> (x+1=w492:dbl)
                      n346 = property on="Yloop" class="DigNum (严格)"("Value"=w492) -> ()  [unwired: 2 in, 2 out]
                    }
                    frame #2 {
                      n347 = property on="Xloop" class="DigNum (严格)"() -> ("Value"=w499:dbl)  [unwired: 2 in, 2 out]
                      n348 = property on="Yloop" class="DigNum (严格)"() -> ("Value"=w496:dbl)  [unwired: 2 in, 2 out]
                      n349 = Initialize Array(0.0 ("元素"), w499, w496) -> (w498:dbl[][])
                      n350 = property on="强度图" class="IntGraph (严格)"("Value"=w498) -> ()  [unwired: 2 in, 2 out]
                    }
                  }
                  n351 = while {
                    shift-right: [w518] -> w478
                    shift-left: w476 -> [w518]
                    stop <- w523 stop-if-true
                    n352 = call "X,Y,Z轴坐标查询.vi"("细分设置"=8.0, "查询坐标轴"="Y", "串口通信端口"=w518) -> ("坐标(mm)"=w525:dbl)
                    n353 = property on="Y起点" class="DigNum (严格)"() -> ("Value"=w517:dbl)  [unwired: 2 in, 2 out]
                    n354 = property on="电机急停" class="Bool (严格)"() -> ("Value"=w524:bool)  [unwired: 2 in, 2 out]
                    n355 = Multiply(x=w525, y=1.0 ("x")) -> (x*y=w521:dbl)
                    n356 = Subtract(x=w517, y=w521) -> (x-y=w520:dbl)
                    n357 = case shown="真" w524 {
                      tunnel: w518 -> [_ w529]
                      frame False {
                      }
                      frame True {
                        n358 = call "步进电机命令输入与输出.vi"("输入字符串"="S0/", "串口通信端口"=w529) -> ()  [unwired: 1 out]
                      }
                    }
                    n359 = Absolute Value(x=w520) -> (abs(x)=w519:dbl)
                    n360 = local read "精度"() -> (w522:dbl)
                    n361 = property on="Y(mm)" class="DigNum (严格)"("Value"=w521) -> ()  [unwired: 2 in, 2 out]
                    n362 = Less?(x=w519, y=w522) -> (x < y?=w523:bool)
                  }
                  n363 = for {
                    N: w475 -> [_]
                    shift-right: [w562] -> _
                    shift-left: w479 -> [w562]
                    shift-right: [w561] -> _
                    shift-left: w482 -> [w561]
                    tunnel: [w560] -> w474 mode=indexing
                    shift-right: [w559] -> w480
                    shift-left: w478 -> [w554]
                    i -> [w555]
                    # "实时成像出问题调这里"
                    n364 = property on="Y序" class="DigNum (严格)"("Value"=w555) -> ()  [unwired: 2 in, 2 out]
                    n365 = flat-sequence {
                      tunnel: w554 -> [w599]
                      tunnel: [w599] -> w558
                      tunnel: [w598] -> w557
                      frame #0 {
                        n366 = property on="X起点" class="DigNum (严格)"() -> ("Value"=w596:dbl)  [unwired: 2 in, 2 out]
                        n367 = property on="细分设置" class="DigNum (严格)"() -> ("Value"=w598:dbl)  [unwired: 2 in, 2 out]
                        n368 = Multiply(x=w596, y=50.0) -> (x*y=w602:dbl)
                        n369 = Multiply(x=w602, y=w598) -> (x*y=w607:dbl)
                        n370 = Tick Count (ms)() -> (millisecond timer value=w595:u32)
                        n371 = local read "等待时间"() -> (w597:u32)
                        n372 = Number To Fractional String(number=w607, precision (6)=i16 0 ("精度(6)")) -> (F-format string=w605:string)  [unwired: 2 out]
                        n373 = property on="time（行）" class="DigNum (严格)"("Value"=w595) -> ()  [unwired: 2 in, 2 out]
                        n374 = Concatenate Strings("X=" ("字符串"), w605, "/" ("字符串")) -> (w600:string)
                        n375 = Wait (ms)(milliseconds to wait=w597) -> ()  [unwired: 1 out]
                        n376 = call "步进电机命令输入与输出.vi"("输入字符串"=w600, "串口通信端口"=w599) -> ()  [unwired: 1 out]
                      }
                    }
                    n377 = while {
                      shift-right: [w610] -> w556
                      shift-left: w558 -> [w610]
                      shift-right: [w608] -> _
                      shift-left: w557 -> [w608]
                      stop <- w614 stop-if-true
                      n378 = property on="电机急停" class="Bool (严格)"() -> ("Value"=w615:bool)  [unwired: 2 in, 2 out]
                      n379 = case shown="真" w615 {
                        tunnel: w610 -> [_ w620]
                        frame False {
                        }
                        frame True {
                          n380 = call "步进电机命令输入与输出.vi"("输入字符串"="S0/", "串口通信端口"=w620) -> ()  [unwired: 1 out]
                        }
                      }
                      n381 = call "X,Y,Z轴坐标查询.vi"("细分设置"=w608, "查询坐标轴"="X", "串口通信端口"=w610) -> ("坐标(mm)"=w616:dbl)
                      n382 = property on="X起点" class="DigNum (严格)"() -> ("Value"=w618:dbl)  [unwired: 2 in, 2 out]
                      n383 = Multiply(x=w616, y=4.0 ("x")) -> (x*y=w612:dbl)
                      n384 = Subtract(x=w618, y=w612) -> (x-y=w611:dbl)
                      n385 = local read "精度"() -> (w613:dbl)
                      n386 = Absolute Value(x=w611) -> (abs(x)=w609:dbl)
                      n387 = property on="X（mm）" class="DigNum (严格)"("Value"=w612) -> ()  [unwired: 2 in, 2 out]
                      n388 = Less?(x=w609, y=w613) -> (x < y?=w614:bool)
                    }
                    n389 = flat-sequence {
                      tunnel: [w625] -> w565
                      tunnel: [w623] -> w564
                      tunnel: [w626] -> w560
                      tunnel: [w624] -> w563
                      tunnel: w556 -> [w622]
                      tunnel: [w661] -> w550
                      tunnel: w561 -> [w641]
                      tunnel: w562 -> [w640]
                      tunnel: w565 -> [w653]
                      tunnel: w564 -> [w661]
                      tunnel: w563 -> [w645]
                      frame #0 {
                        n390 = local read "精度"() -> (w634:dbl)
                        n391 = property on="细分设置" class="DigNum (严格)"() -> ("Value"=w633:dbl)  [unwired: 2 in, 2 out]
                        n392 = property on="X终点" class="DigNum (严格)"() -> ("Value"=w637:dbl)  [unwired: 2 in, 2 out]
                        n393 = local read "pulDDR2Length"() -> (w629:u32)
                        n394 = local read "M_Length"() -> (w631:i32)
                        n395 = property on="hDevice" class="DigNum (严格)"() -> ("Value"=w630:i32)  [unwired: 2 in, 2 out]
                        n396 = property on="N_Length" class="DigNum (严格)"() -> ("Value"=w632:i32)  [unwired: 2 in, 2 out]
                        n397 = property on="等待时间" class="DigNum (严格)"() -> ("Value"=w635:u32)  [unwired: 2 in, 2 out]
                        n398 = property on="电机急停" class="Bool (严格)"() -> ("Value"=w636:bool)  [unwired: 2 in, 2 out]
                        n399 = call "X轴连续扫描（初稿）.vi"("VISA I"=w622, "X"=w637, "精度"=w634, "细分设置"=w633, "等待时间(ms)"=w635, "pulDDR2Length"=w629, "电机急停"=w636, "hDevice"=w630, "M-length"=w631, "N-length"=w632) -> ("VISA O"=w623:refnum<visa-resource-name>, "hDevice out"=w628:i32, "X"=w627:dbl, "强度图行"=w626:dbl[], "时域谱页"=w625:dbl[][], "幅频谱页"=w624:dbl[][])  [unwired: 4 in]
                        n400 = property on="hDevice 2" class="DigNum (严格)"("Value"=w628) -> ()  [unwired: 2 in, 2 out]
                        n401 = property on="X（mm）" class="DigNum (严格)"("Value"=w627) -> ()  [unwired: 2 in, 2 out]
                      }
                      frame #1 {
                        n402 = local read "time（行）"() -> (w660:u32)
                        n403 = Tick Count (ms)() -> (millisecond timer value=w657:u32)
                        n404 = Subtract(x=w657, y=w660) -> (x-y=w659:u32)
                        n405 = property on="Y序" class="DigNum (严格)"() -> ("Value"=w638:i32)  [unwired: 2 in, 2 out]
                        n406 = Multiply(x=w659, y=0.001) -> (x*y=w639:dbl)
                        n407 = property on="行用时（s）" class="DigNum (严格)"("Value"=w639) -> ()  [unwired: 2 in, 2 out]
                        n408 = Increment(x=w638) -> (x+1=w642:i32)
                        n409 = Number To Decimal String(number=w642) -> (decimal integer string=w651:string)  [unwired: 1 in]
                        n410 = Number To Decimal String(number=w642) -> (decimal integer string=w650:string)  [unwired: 1 in]
                        n411 = Concatenate Strings("T" ("字符串"), w651, ".txt" ("字符串")) -> (w654:string)
                        n412 = Concatenate Strings("F" ("字符串"), w650, ".txt" ("字符串")) -> (w648:string)
                        n413 = Build Path(base path=w641, name or relative path=w654) -> (appended path=w656:path)
                        n414 = call-poly <vilib>:"Write Delimited Spreadsheet.vi"("file path (dialog if empty)"=w656, "2D data"=w653, "transpose? (no:F)"=FALSE) -> ()  [unwired: 11 in, 2 out]
                        n415 = Build Path(base path=w640, name or relative path=w648) -> (appended path=w646:path)
                        n416 = call-poly <vilib>:"Write Delimited Spreadsheet.vi"("file path (dialog if empty)"=w646, "2D data"=w645, "transpose? (no:F)"=FALSE) -> ()  [unwired: 11 in, 2 out]
                      }
                    }
                    n417 = flat-sequence {
                      tunnel: w550 -> [w572]
                      tunnel: [w572] -> w551
                      tunnel: [w571] -> w552
                      frame #0 {
                        n418 = property on="细分设置" class="DigNum (严格)"() -> ("Value"=w571:dbl)  [unwired: 2 in, 2 out]
                        n419 = Multiply(x=0.0, y=50.0) -> (x*y=w575:dbl)
                        n420 = Multiply(x=w575, y=w571) -> (x*y=w580:dbl)
                        n421 = local read "等待时间"() -> (w570:u32)
                        n422 = Number To Fractional String(number=w580, precision (6)=i16 0 ("精度(6)")) -> (F-format string=w578:string)  [unwired: 2 out]
                        n423 = Concatenate Strings("X=" ("字符串"), w578, "/" ("字符串")) -> (w573:string)
                        n424 = Wait (ms)(milliseconds to wait=w570) -> ()  [unwired: 1 out]
                        n425 = call "步进电机命令输入与输出.vi"("输入字符串"=w573, "串口通信端口"=w572) -> ()  [unwired: 1 out]
                      }
                    }
                    n426 = while {
                      shift-right: [w584] -> w549
                      shift-left: w551 -> [w584]
                      shift-right: [w582] -> _
                      shift-left: w552 -> [w582]
                      stop <- w588 stop-if-true
                      n427 = property on="电机急停" class="Bool (严格)"() -> ("Value"=w589:bool)  [unwired: 2 in, 2 out]
                      n428 = case shown="真" w589 {
                        tunnel: w584 -> [_ w593]
                        frame False {
                        }
                        frame True {
                          n429 = call "步进电机命令输入与输出.vi"("输入字符串"="S0/", "串口通信端口"=w593) -> ()  [unwired: 1 out]
                        }
                      }
                      n430 = call "X,Y,Z轴坐标查询.vi"("细分设置"=w582, "查询坐标轴"="X", "串口通信端口"=w584) -> ("坐标(mm)"=w590:dbl)
                      n431 = Multiply(x=w590, y=4.0 ("x")) -> (x*y=w586:dbl)
                      n432 = Subtract(x=0.0, y=w586) -> (x-y=w585:dbl)
                      n433 = local read "精度"() -> (w587:dbl)
                      n434 = Absolute Value(x=w585) -> (abs(x)=w583:dbl)
                      n435 = property on="X（mm）" class="DigNum (严格)"("Value"=w586) -> ()  [unwired: 2 in, 2 out]
                      n436 = Less?(x=w583, y=w587) -> (x < y?=w588:bool)
                    }
                    n437 = property on="强度图" class="IntGraph (严格)"() -> ("Value"=w568:dbl[][])  [unwired: 2 in, 2 out]
                    n438 = property on="Yloop" class="DigNum (严格)"() -> ("Value"=w547:dbl)  [unwired: 2 in, 2 out]
                    n439 = property on="Y序" class="DigNum (严格)"() -> ("Value"=w553:i32)  [unwired: 2 in, 2 out]
                    n440 = Replace Array Subset(array=w568, new element=w560, index (col)=w553) -> (w567:dbl[][])  [unwired: 1 in]
                    n441 = property on="强度图" class="IntGraph (严格)"("Value"=w567) -> ()  [unwired: 2 in, 2 out]
                    n442 = Decrement(x=w547) -> (x-1=w548:dbl)
                    n443 = Equal?(x=w553, y=w548) -> (x = y?=w566:bool)
                    n444 = case shown="真" w566 {
                      tunnel: w549 -> [w665 w695]
                      tunnel: [w663 w696] -> w559
                      frame False {
                        n445 = flat-sequence {
                          tunnel: w665 -> [w669]
                          tunnel: [w669] -> w664
                          tunnel: [w666] -> w662
                          frame #0 {
                            n446 = property on="细分设置" class="DigNum (严格)"() -> ("Value"=w666:dbl)  [unwired: 2 in, 2 out]
                            n447 = call "X,Y,Z轴坐标查询.vi"("细分设置"=w666, "查询坐标轴"="Y", "串口通信端口"=w669) -> ("坐标(mm)"=w670:dbl)
                            n448 = property on="Y:" class="DigNum (严格)"() -> ("Value"=w668:dbl)  [unwired: 2 in, 2 out]
                            n449 = Add(x=w670, y=w668) -> (x+y=w672:dbl)
                            "x+y 3" <- w672
                            n450 = Multiply(x=w672, y=200.0) -> (x*y=w676:dbl)
                            n451 = Multiply(x=w676, y=8.0 ("细分设置")) -> (x*y=w681:dbl)
                            n452 = Number To Fractional String(number=w681, precision (6)=i16 0 ("精度(6)")) -> (F-format string=w679:string)  [unwired: 2 out]
                            n453 = Concatenate Strings("Y=" ("字符串"), w679, "/" ("字符串")) -> (w674:string)
                            n454 = call "步进电机命令输入与输出.vi"("输入字符串"=w674, "串口通信端口"=w669) -> ()  [unwired: 1 out]
                            n455 = property on="等待时间" class="DigNum (严格)"() -> ("Value"=w667:u32)  [unwired: 2 in, 2 out]
                            n456 = Wait (ms)(milliseconds to wait=w667) -> ()  [unwired: 1 out]
                          }
                        }
                        n457 = while {
                          shift-right: [w684] -> w663
                          shift-left: w664 -> [w684]
                          shift-right: [w683] -> _
                          shift-left: w662 -> [w683]
                          stop <- w690 stop-if-true
                          n458 = call "X,Y,Z轴坐标查询.vi"("细分设置"=w683, "查询坐标轴"="Y", "串口通信端口"=w684) -> ("坐标(mm)"=w688:dbl)
                          n459 = property on="x+y 3" class="DigNum (严格)"() -> ("Value"=w682:dbl)  [unwired: 2 in, 2 out]
                          n460 = property on="电机急停" class="Bool (严格)"() -> ("Value"=w687:bool)  [unwired: 2 in, 2 out]
                          n461 = property on="Y(mm)" class="DigNum (严格)"("Value"=w688) -> ()  [unwired: 2 in, 2 out]
                          n462 = case shown="真" w687 {
                            tunnel: w684 -> [_ w692]
                            frame False {
                            }
                            frame True {
                              n463 = call "步进电机命令输入与输出.vi"("输入字符串"="S0/", "串口通信端口"=w692) -> ()  [unwired: 1 out]
                            }
                          }
                          n464 = Subtract(x=w682, y=w688) -> (x-y=w686:dbl)
                          n465 = Absolute Value(x=w686) -> (abs(x)=w685:dbl)
                          n466 = local read "精度"() -> (w689:dbl)
                          n467 = Less?(x=w685, y=w689) -> (x < y?=w690:bool)
                        }
                      }
                      frame True {
                        n468 = flat-sequence {
                          tunnel: [w700] -> _
                          tunnel: [w700] -> w697
                          tunnel: w695 -> [w700]
                          tunnel: [w698] -> w694
                          frame #0 {
                            n469 = property on="细分设置" class="DigNum (严格)"() -> ("Value"=w698:dbl)  [unwired: 2 in, 2 out]
                            n470 = Multiply(x=0.0, y=200.0) -> (x*y=w704:dbl)
                            n471 = Multiply(x=w704, y=w698) -> (x*y=w709:dbl)
                            n472 = Number To Fractional String(number=w709, precision (6)=i16 0 ("精度(6)")) -> (F-format string=w707:string)  [unwired: 2 out]
                            n473 = Concatenate Strings("Y=" ("字符串"), w707, "/" ("字符串")) -> (w702:string)
                            n474 = call "步进电机命令输入与输出.vi"("输入字符串"=w702, "串口通信端口"=w700) -> ()  [unwired: 1 out]
                            n475 = property on="等待时间" class="DigNum (严格)"() -> ("Value"=w699:u32)  [unwired: 2 in, 2 out]
                            n476 = Wait (ms)(milliseconds to wait=w699) -> ()  [unwired: 1 out]
                          }
                        }
                        n477 = while {
                          shift-right: [w711] -> w696
                          shift-left: w697 -> [w711]
                          shift-right: [w710] -> _
                          shift-left: w694 -> [w710]
                          stop <- w717 stop-if-true
                          n478 = property on="电机急停" class="Bool (严格)"() -> ("Value"=w718:bool)  [unwired: 2 in, 2 out]
                          n479 = call "X,Y,Z轴坐标查询.vi"("细分设置"=w710, "查询坐标轴"="Y", "串口通信端口"=w711) -> ("坐标(mm)"=w719:dbl)
                          n480 = case shown="真" w718 {
                            tunnel: w711 -> [_ w722]
                            frame False {
                            }
                            frame True {
                              n481 = call "步进电机命令输入与输出.vi"("输入字符串"="S0/", "串口通信端口"=w722) -> ()  [unwired: 1 out]
                            }
                          }
                          n482 = Multiply(x=w719, y=1.0 ("x")) -> (x*y=w715:dbl)
                          n483 = Subtract(x=w715, y=0.0 ("x")) -> (x-y=w713:dbl)
                          n484 = local read "精度"() -> (w716:dbl)
                          n485 = Absolute Value(x=w713) -> (abs(x)=w712:dbl)
                          n486 = property on="Y(mm)" class="DigNum (严格)"("Value"=w715) -> ()  [unwired: 2 in, 2 out]
                          n487 = Less?(x=w712, y=w716) -> (x < y?=w717:bool)
                        }
                      }
                    }
                  }
                  n488 = flat-sequence {
                    tunnel: [w531] -> _
                    tunnel: w474 -> [w532]
                    tunnel: [w531] -> w481
                    tunnel: w480 -> [w531]
                    frame #0 {
                      n489 = local read "毫秒计时值"() -> (w537:u32)
                      n490 = property on="数组" class="Arr (严格)"("Value"=w532) -> ()  [unwired: 2 in, 2 out]
                      n491 = Transpose 2D Array(2D array=w532) -> (transposed array=w534:dbl[][])
                      n492 = Tick Count (ms)() -> (millisecond timer value=w538:u32)
                      n493 = property on="强度图" class="IntGraph (严格)"("Value"=w534) -> ()  [unwired: 2 in, 2 out]
                      n494 = Subtract(x=w538, y=w537) -> (x-y=w535:u32)
                      n495 = Multiply(x=w535, y=0.001) -> (x*y=w533:dbl)
                      n496 = property on="总用时（s）" class="DigNum (严格)"("Value"=w533) -> ()  [unwired: 2 in, 2 out]
                    }
                  }
                }
                event "分层图查看": Value Change {
                  n497 = event-data() -> ()  [unwired: 1 in, 6 out]
                  n498 = call "分层图显示1.1.vi"("IN"=w725) -> ("OUT"=w724:string)  [unwired: 10 in]
                }
              }
            }
          }
        }
        n499 = dll-call lib="PTH2]abs CUsersH301Desktopart闭环扫描程序采集卡控制INFamd64\nPCI8502_32" fn="PCI8502_ReleaseDeviceAD" label="ReleaseDeviceAD"("hDevice"="hDevice 2") -> ("hDevice"=w23:i32)  [unwired: 4 in, 2 out]
        n500 = VISA Close(VISA resource name=w21) -> (error out=→"错误输出":errorcluster)  [unwired: 1 in]
        n501 = dll-call lib="PTH2]abs CUsersH301Desktopart闭环扫描程序采集卡控制INFamd64\nPCI8502_32" fn="PCI8502_ReleaseDevice" label="ReleaseDevice"("hDevice"=w23) -> ()  [unwired: 5 in, 2 out]
        "M_Length" <- w27
      }
    }
  }
  n502 = property on="高级设置" class="Bool"("Visible"=FALSE ("可见")) -> ()  [unwired: 2 in, 2 out]
  n503 = property on="定位模式" class="Bool"("Visible"=FALSE ("可见")) -> ()  [unwired: 2 in, 2 out]
